vi "no result query test.vi"() -> ()   [LabVIEW 2020, in "mysql.lvlib" / "mysql.lvclass"]
uses:
  mysql.net/mysql.lvclass
  456c3c5f-9dac-4558-bbbd-4e5e7f663426.vi
  <vilib>/Utility/error.llb/Error Cluster From Error Code.vi
panel:
  in  "Connection string":string="server=127.0.0.1;uid=root;pwd=Jazz@422521;database=test"
  in  "error in (no error)":errorcluster
  out "error out":errorcluster={"status"=TRUE, "code"=1172, "source"="Invoke Node System.Reflection.TargetInvocationException: Exception has been thrown by the target of an invocation.\n\tInner Exception: System.InvalidOperationException: Connection must be valid and open. <append><b>System.InvalidOperationException</b> in mysql.lvlib:mysql.lvclass:Query.vi->mysql.lvlib:mysql.lvclass:no result query test.vi"}
  in  "Query string":string="CREATE TABLE animals (\n     id MEDIUMINT NOT NULL AUTO_INCREMENT,\n     name CHAR(30) NOT NULL,\n     PRIMARY KEY (id)\n);\nINSERT INTO animals (name) VALUES\n    ('dog'),('cat'),('penguin'),\n    ('lax'),('whale'),('ostrich');"
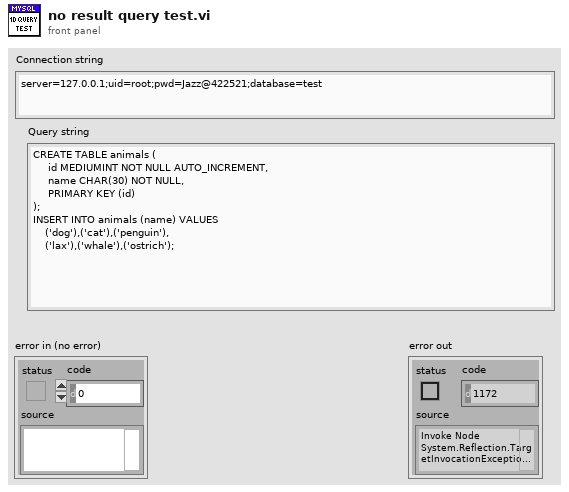
[diagram p1: front panel]
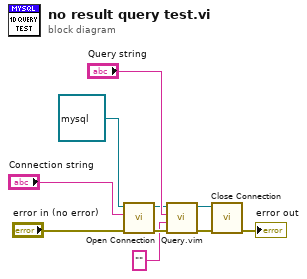
[diagram p0: block diagram]
diagram:
  n1 = call-dynamic "Open Connection.vi"("error in (no error)"="error in (no error)", "Connection string"="Connection string", "mysql in"=refnum<class "mysql.lvclass"> refnum) -> ("error out"=w2:errorcluster, "mysql out"=w3:refnum<class "mysql.lvclass">)  [unwired: 7 in]
  n2 = call "Query.vim"("error in (no error)"=w2, "Type and Default"="", "Query string"="Query string", "IDatabase in"=w3) -> ("error out"=w9:errorcluster, "IDatabase out"=w10:refnum<class "mysql.lvclass">)  [unwired: 5 in, 1 out]
  n3 = call-dynamic "Close Connection.vi"("error in (no error)"=w9, "mysql in"=w10) -> ("error out"=→"error out":errorcluster)  [unwired: 8 in, 1 out]
